vi "Write Digital Pattern Generator Resource Name.vi"(10 "Digital Pattern Generator Resource Name":refnum<k15>="HSD_6570_C1_S02" caption="resource name", 11 "niDigital in":refnum<class "niDigital.lvclass">) -> (3 "niDigital out":refnum<class "niDigital.lvclass">)   [LabVIEW 2020, in "niDigital.lvclass"]
uses:
  niDigital.lvclass
  niDigital.lvclass/niDigital.ctl
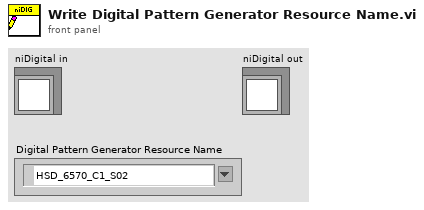
[diagram p1: front panel]
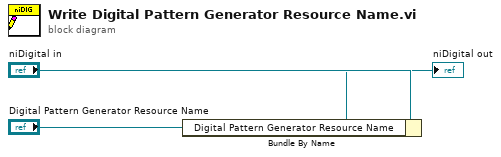
[diagram p0: block diagram]
diagram:
  n1 = Bundle By Name(cluster="niDigital in", "Digital Pattern Generator Resource Name"="Digital Pattern Generator Resource Name") -> (→"niDigital out":refnum<class "niDigital.lvclass">)
